vi "Set Sweep.vi"(4 "sweep type (0 : linear)":T1, 6 "Number of Points":i32, 8 "error in (no error)":errorcluster, 9 "Stop (Hz)":dbl, 10 "Start (Hz)":dbl, 11 "Instrument.VSource in":refnum<class "Instrument.VNA.lvclass">) -> (0 "error out":errorcluster, 3 "Instrument.VSource out":refnum<class "Instrument.VNA.lvclass">)   [LabVIEW 2020, in "Instrument.VNA.lvclass"]
uses:
  Instrument.VNA.lvclass
  Typedefs/Sweep Type--enum.ctl
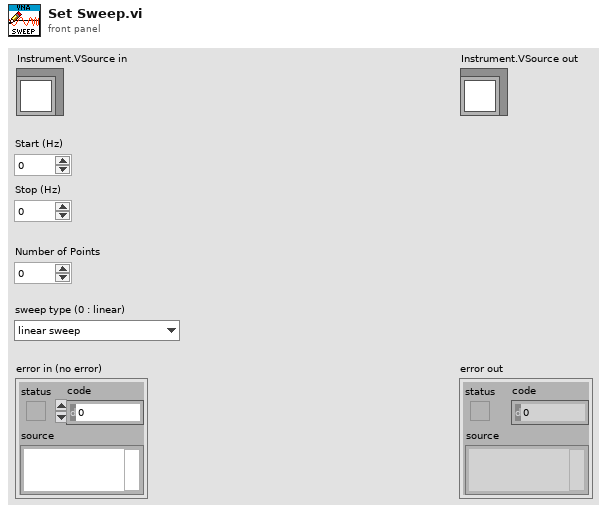
[diagram p1: front panel]
types:
  T1 = typedef "Instrument.VNA.lvclass/Sweep Type--enum.ctl" = enum16{"linear sweep", "logarithmic sweep", "frequency list", "CW time sweep", "power sweep"}
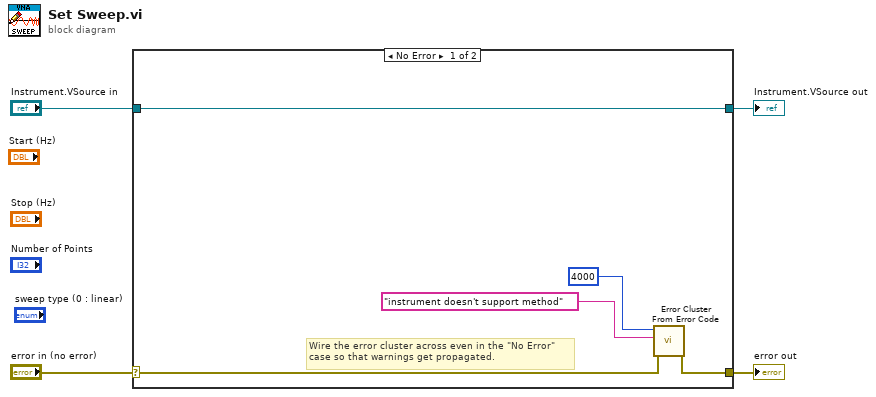
[diagram p0: block diagram]
diagram:
  n1 = case shown="No Error" "error in (no error)" {
    selector: "error in (no error)" -> [w6 w11]
    tunnel: [w5 w11] -> w3
    tunnel: [w9 w10] -> w1
    tunnel: "Instrument.VSource in" -> [w9 w10]
    frame No Error {
      # "Wire the error cluster across even in the \"No Error\"\ncase so that warnings get propagated."
      n2 = call <vilib>:"Error Cluster From Error Code.vi"("error in (no error)"=w6, "error message (\"\")"="instrument doesn't support method" ("error message (\"\")"), "error code (0)"=4000) -> ("error out"=w5:errorcluster)  [unwired: 6 in]
    }
    frame Error {
    }
  }
  "error out" <- w3
  "Instrument.VSource out" <- w1
